vi "init.vi"(8 "error in":errorcluster, 10 "TBM module configuration in":refnum<class "TBM module configuration.lvclass">, 11 "Profibus Module runtime in":refnum<class "Profibus Module runtime.lvclass">) -> (0 "error out":errorcluster, 1 "data allocations":T1, 2 "execution settings":T4, 3 "Profibus Module runtime out":refnum<class "Profibus Module runtime.lvclass">)   [LabVIEW 2013, in "Profibus Module runtime.lvclass"]
doc: "Provides an interface for initializing a module at runtime. While this interface performs no operations, a child should provide an override which may open any necessary references or sessions, allocate necessary memory, and perform any final configuration validataion before providing the full configuration <b>execution data</b> to the calling process."
uses:
  Profibus Module runtime.lvclass
  <vilib>/NI/Tag Bus Module Framework/module configuration/TBM module configuration.lvclass
  <vilib>/NI/Tag Bus Module Framework/runtime/execution settings.ctl
  <vilib>/NI/Tag Bus Module Framework/channel/data tables.ctl
  <vilib>/NI/Tag Bus/dictionary/data dictionary.lvclass
  <vilib>/NI/Tag Bus/dictionary table pair.ctl
  <vilib>/NI/Tag Bus/table/data table.ctl
  configuration/Profibus Module configuration.lvclass
  dynamic profibus/fpga reference.ctl
  <vilib>/NI/Tag Bus Module Framework/FPGA manager/methods.ctl
  configuration/Profibus Module configuration.lvclass/Profibus Module configuration.ctl
  channel/Profibus channel.lvclass
  channel/Profibus channel.lvclass/Profibus channel.ctl
  Profibus Module runtime.lvclass/Profibus Module runtime.ctl
  <vilib>/NI/Tag Bus Module Framework/channel/TBM channel.lvclass
  <vilib>/NI/Tag Bus Module Framework/runtime/TBM module execution interface.lvclass
  dynamic profibus/dynamic profibus.lvlib
  <vilib>/NI/Tag Bus Module Framework/FPGA manager/FPGA manager.lvlib
  <vilib>/NI/Tag Bus/tag bus.lvlib
  <vilib>/NI/Tag Bus/table/data table.lvlib
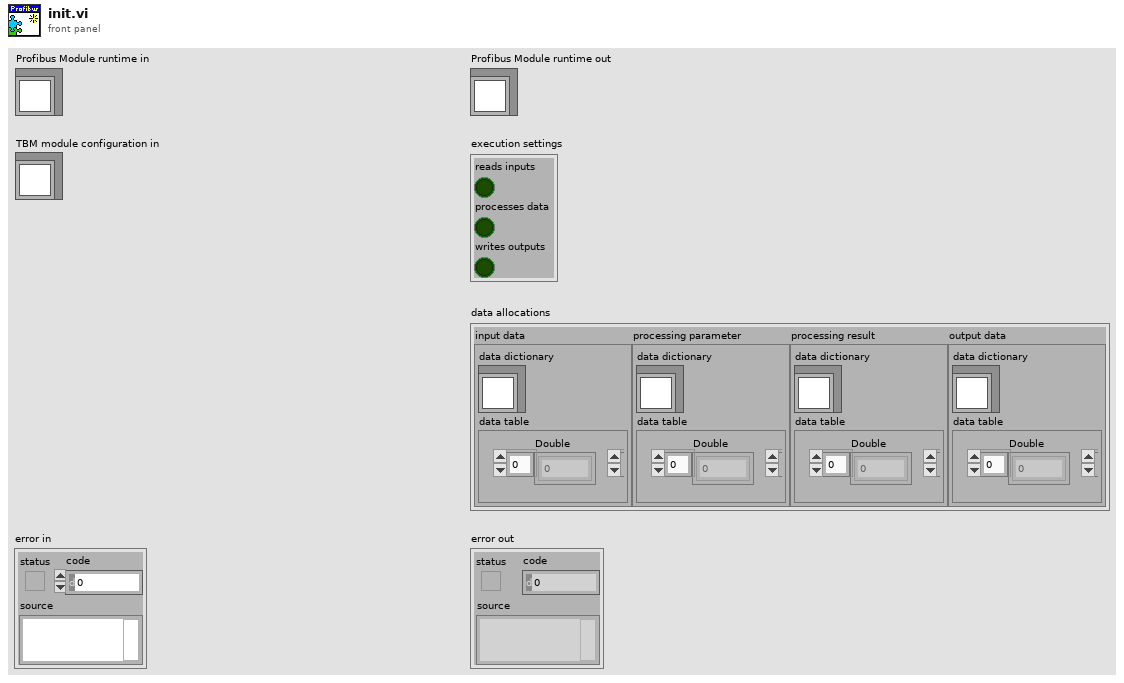
[diagram p1: front panel]
types:
  T1 = typedef "TBM channel.lvclass/data tables.ctl" = cluster{"input data":T2, "processing parameter":T2, "processing result":T2, "output data":T2}
  T2 = typedef "tag bus.lvlib/dictionary table pair.ctl" = cluster{"data dictionary":refnum<class "data dictionary.lvclass">, "data table":T3}
  T3 = typedef "tag bus.lvlib/data table.lvlib/data table.ctl" = cluster{"Double":dbl[], "Single":sgl[], "I64":i64[], "I32":i32[], "I16":i16[], "I8":i8[], "U64":u64[], "U32":u32[], "U16":u16[], "U8":u8[], "Boolean":bool[], "String":string[], "Array of Double":cluster{"DBL Array":dbl[]}[], "Array of Single":cluster{"SGL Array":sgl[]}[], "Array of I64":cluster{"I64 Array":i64[]}[], "Array of I32":cluster{"I32 Array":i32[]}[], "Array of I16":cluster{"I16 Array":i16[]}[], "Array of I8":cluster{"I8 Array":i8[]}[], "Array of U64":cluster{"U64 Array":u64[]}[], "Array of U32":cluster{"U32 Array":u32[]}[], "Array of U16":cluster{"U16 Array":u16[]}[], "Array of U8":cluster{"U8 Array":u8[]}[], "Array of Boolean":cluster{"Boolean Array":bool[]}[], "Array of String":cluster{"String Array":string[]}[]}
  T4 = typedef "TBM module execution interface.lvclass/execution settings.ctl" = cluster{"reads inputs":bool, "processes data":bool, "writes outputs":bool}
  T5 = typedef "FPGA manager.lvlib/methods.ctl" = enum16{"initialize bitfile", "cache bitfile", "locate bitfile", "close bitfile", "clear manager"}
  T6 = typedef "dynamic profibus.lvlib/fpga reference.ctl" = refnum<k20>
  T7 = cluster{"Address":i8, "Input Length":u8, "Output Length":u8}[]
  T8 = typedef "Profibus Module runtime.lvclass/profibus diagnostics reporting.ctl" = cluster{"slave":i8, "report":bool, "diagnostic tag":i32, "error specs":T9[], "buffer":u8[], "true length":u8}
  T9 = typedef "Profibus Module configuration.lvclass/error throw specification.ctl" = cluster{"byte":i32, "bit":i32, "inverted?":bool, "error":i32}
  T10 = typedef "Profibus Module runtime.lvclass/profibus slave configuration.ctl" = cluster{"slave index":i8, "data items":T11[], "data buffer":u8[], "big endian":bool, "command list":u32[], "data offset":u8}
  T11 = typedef "Profibus Module runtime.lvclass/profibus mapping configuration.ctl" = cluster{"data type":T12, " byte":i32, " bit":i32, "tag index":i32}
  T12 = typedef "tag bus.lvlib/tag descriptor.lvclass/Data Type.ctl" = enum16{"Double", "Single", "I64", "I32", "I16", "I8", "U64", "U32", "U16", "U8", "Boolean", "String", "Array of Double", "Array of Single", "Array of I64", "Array of I32", "Array of I16", "Array of I8", "Array of U64", "Array of U32", "Array of U16", "Array of U8", "Array of Boolean", "Array of String"}
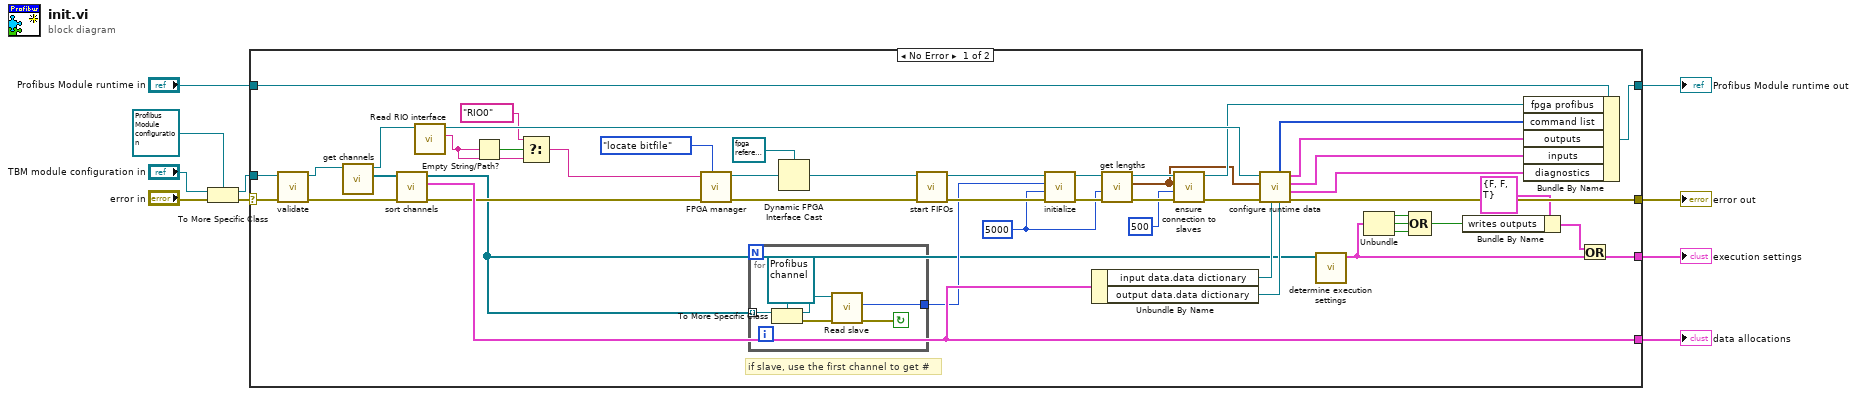
[diagram p0: block diagram]
diagram:
  n1 = To More Specific Class(target class=refnum<class "Profibus Module configuration.lvclass"> refnum ("Synchronous module configuration"), reference="TBM module configuration in", error in="error in") -> (specific class reference=w9:refnum<class "Profibus Module configuration.lvclass">, error out=w10:errorcluster)
  n2 = case shown="No Error" w10 {
    selector: w10 -> [w56 w65]
    tunnel: w9 -> [w55 _]
    tunnel: "Profibus Module runtime in" -> [w58 w66]
    tunnel: [w52 w66] -> w4
    tunnel: [w49 w65] -> w3
    tunnel: [w48 _] -> w1
    tunnel: [w28 _] -> w2
    frame No Error {
      w18 = 5000 ("Timeout (ms)")
      # "if slave, use the first channel to get #"
      n3 = call-dynamic "validate.vi"("error in"=w56, "Profibus Module configuration in"=w55) -> ("error out"=w57:errorcluster, "Profibus Module configuration out"=w54:refnum<class "Profibus Module configuration.lvclass">)  [unwired: 8 in]
      n4 = call-dynamic "get channels.vi"("Profibus Module configuration in"=w54) -> ("channels"=w53:refnum<class "TBM channel.lvclass">[], "Profibus Module configuration out"=w44:refnum<class "Profibus Module configuration.lvclass">)  [unwired: 9 in]
      n5 = call <vilib>:"sort channels.vi"("error in"=w57, "channels in"=w53) -> ("error out"=w40:errorcluster, "data allocations"=w48:T1, "channels out"=w24:refnum<class "TBM channel.lvclass">[])  [unwired: 7 in]
      n6 = call "Read RIO interface.vi"("Profibus Module configuration in"=w44) -> ("RIO interface"=w41:string, "Profibus Module configuration out"=w45:refnum<class "Profibus Module configuration.lvclass">)  [unwired: 8 in, 1 out]
      n7 = Empty String/Path?(string/path=w41) -> (empty?=w43:bool)
      n8 = Select(t=tag "RIO0" ("resource name"), s=w43, f=w41) -> (s? t:f=w38:string)
      n9 = call <vilib>:"FPGA manager.vi"("action"=methods."locate bitfile", "error in"=w40, "RIO resource"=w38) -> ("error out"=w26:errorcluster, "bitfile"=w39:refnum<k20>)  [unwired: 6 in, 1 out]
      n10 = for {
        tunnel: [w61] -> w25
        tunnel: w24 -> [w60] mode=indexing
        stop <- w59 continue-if-true
        n11 = To More Specific Class(target class=refnum<class "Profibus channel.lvclass"> refnum ("Profibus channel in"), reference=w60) -> (specific class reference=w63:refnum<class "Profibus channel.lvclass">, error out=w64:errorcluster)  [unwired: 1 in]
        n12 = call "Read slave.vi"("error in"=w64, "Profibus channel in"=w63) -> ("error out"=w59:errorcluster, "slave"=w61:i8)  [unwired: 7 in, 1 out]
      }
      n13 = Dynamic FPGA Interface Cast(Session In=T6 refnum ("profibus reference"), Type=w39) -> (Session Out=w30:T6)
      n14 = call "start FIFOs.vi"("error in"=w26, "profibus reference"=w30) -> ("error out"=w31:errorcluster, "profibus reference out"=w29:T6)  [unwired: 8 in]
      n15 = call "initialize.vi"("error in"=w31, "Timeout (ms)"=w18, "device (if slave)"=w25, "profibus reference"=w29) -> ("error out"=w35:errorcluster, "profibus reference out"=w34:T6)  [unwired: 6 in]
      n16 = Unbundle By Name(w48) -> ("input data.data dictionary"=w32:refnum<class "data dictionary.lvclass">, "output data.data dictionary"=w47:refnum<class "data dictionary.lvclass">)
      n17 = call "get lengths.vi"("error in"=w35, "Timeout (ms)"=w18, "profibus reference"=w34) -> ("error out"=w21:errorcluster, "Slave Info List"=w19:T7, "profibus reference out"=w23:T6)  [unwired: 6 in]
      n18 = call "ensure connection to slaves.vi"("error in"=w21, "Timeout (ms)"=500, "Slave Info List"=w19, "profibus reference"=w23) -> ("error out"=w20:errorcluster, "profibus reference out"=w22:T6)  [unwired: 6 in]
      n19 = call "configure runtime data.vi"("output dictionary"=w47, "input dictionary"=w32, "error in"=w20, "Slave Info List"=w19, "Profibus Module configuration in"=w45) -> ("error out"=w49:errorcluster, "diagnostics"=w36:T8[], "inputs"=w50:T10[], "outputs"=w51:T10[], "full command list"=w33:u32[])  [unwired: 2 in]
      n20 = call <vilib>:"determine execution settings.vi"("channels"=w24) -> ("execution settings"=w16:T4)  [unwired: 10 in]
      n21 = Unbundle(w16) -> ("reads inputs"=w13:bool, "processes data"=w14:bool, "writes outputs"=w15:bool)
      n22 = Compound Arithmetic op=OR(w13, w14, w15) -> (w11:bool)
      n23 = Bundle By Name(cluster=T4 {"reads inputs"=FALSE, "processes data"=FALSE, "writes outputs"=TRUE} ("x"), "writes outputs"=w11) -> (w12:T4)
      n24 = Bundle By Name(cluster=w58, "fpga profibus"=w22, "command list"=w33, "outputs"=w51, "inputs"=w50, "diagnostics"=w36) -> (w52:refnum<class "Profibus Module runtime.lvclass">)
      n25 = Or(x=w12, y=w16) -> (x .or. y?=w28:T4)
    }
    frame Error {
    }
  }
  "error out" <- w3
  "Profibus Module runtime out" <- w4
  "execution settings" <- w2
  "data allocations" <- w1
